vi "main_create_environment.vi"(3 "Meth. Path":refnum<vi>, 4 "Hydr. Path":refnum<vi>, 5 "Ready?":refnum<vi>, 6 "Storage?":refnum<vi>, 7 "Methane?":refnum<vi>, 8 "Running?":refnum<vi>, 9 "Directory":refnum<vi>, 10 "Create":refnum<vi>, 11 "Environtment Tree":refnum<vi>) -> ()   [LabVIEW 2019]
uses:
  lib/libSimulationControl/libSimulationControl.lvlib
panel:
  # "*******************************************************************\nBiogas Plant Control\n\nAuthor: Paul Zügel\nGCSC-Frankfurt am Main 2020\n\n*******************************************************************"
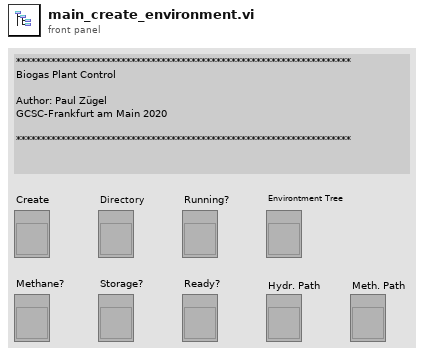
[diagram p1: front panel]
types:
  T1 = cluster{"filename without extension":string, "Child Text":string[], "Child Tag":string, i32, "Child Only?":bool, "Glyph Index":i32}[]
  T2 = enum8{"Enabled", "Disabled", "Disabled and Grayed Out"}
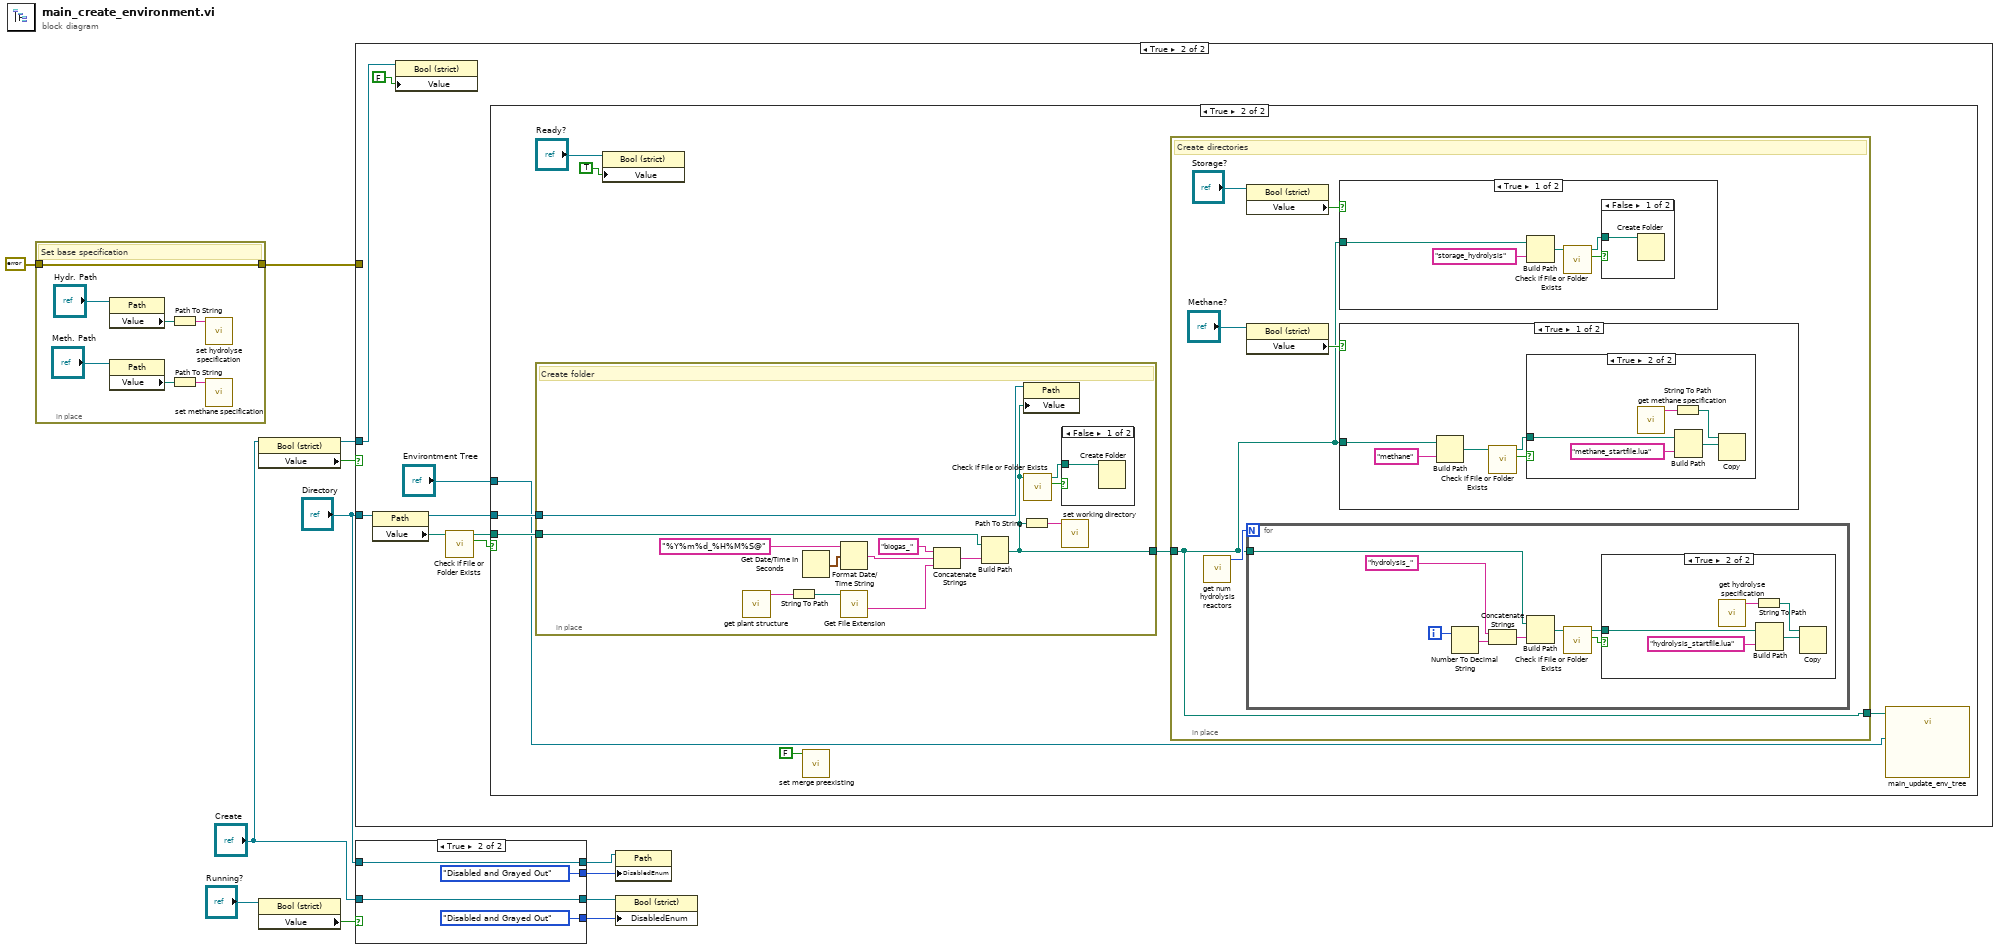
[diagram p0: block diagram]
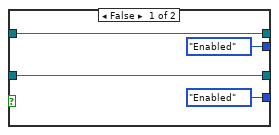
[diagram p2: hidden frame]
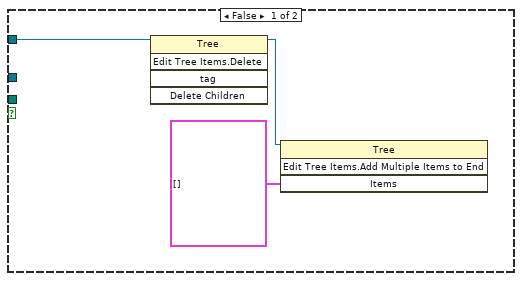
[diagram p4: hidden frame]
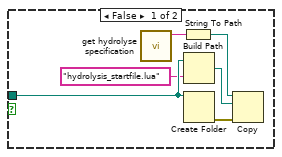
[diagram p6: hidden frame]
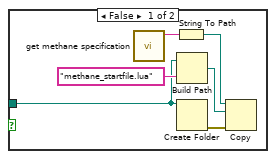
[diagram p7: hidden frame]
diagram:
  n1 = in-place {
    in-place-border: errorcluster {"status"=FALSE, "code"=0, "source"=""} ("error constant") -> [w13]
    in-place-border: [w13] -> w1
    # "Set base specification"
    n2 = property class="Path"(reference="Hydr. Path") -> ("Value"=w15:path)  [unwired: 1 in, 2 out]
    n3 = property class="Path"(reference="Meth. Path") -> ("Value"=w18:path)  [unwired: 1 in, 2 out]
    n4 = Path To String(path=w15) -> (string=w14:string)
    n5 = Path To String(path=w18) -> (string=w17:string)
    n6 = call "set hydrolyse specification.vi"("hydrolyse_spec_file"=w14) -> ()  [unwired: 10 in, 1 out]
    n7 = call "set methane specification.vi"("methane_spec_file"=w17) -> ()  [unwired: 10 in, 1 out]
  }
  n8 = property class="Bool (strict)"(reference="Create") -> (reference out=w11:refnum<vi>, "Value"=w12:bool)  [unwired: 1 in, 1 out]
  n9 = property on="Property Node" class="Bool (strict)"(reference="Running?") -> ("Value"=w9:bool)  [unwired: 1 in, 2 out]
  n10 = case shown="True" w12 {
    tunnel: w11 -> [_ w24]
    tunnel: "Directory" -> [_ w22]
    tunnel: w1 -> [_ _]
    frame False {
    }
    frame True {
      n11 = property class="Path"(reference=w22) -> (reference out=w21:refnum<vi>, "Value"=w25:path)  [unwired: 1 in, 1 out]
      n12 = property class="Bool (strict)"(reference=w24, "Value"=FALSE) -> ()  [unwired: 1 in, 2 out]
      n13 = call <vilib>:"Check if File or Folder Exists.vi"("path"=w25) -> ("file or folder exists?"=w27:bool, "dup path"=w26:path)  [unwired: 8 in, 1 out]
      n14 = case shown="True" w27 {
        tunnel: w26 -> [_ w38]
        tunnel: w21 -> [_ w34]
        tunnel: "Environtment Tree" -> [w28 w31]
        frame False {
          n15 = invoke class="Tree" method="Edit Tree Items.Delete"(reference=w28) -> (reference out=w29:refnum<vi>)  [unwired: 4 in, 4 out]
          n16 = invoke on="Invoke Node" class="Tree" method="Edit Tree Items.Add Multiple Items to End"(reference=w29, "Items"=T1 []) -> ()  [unwired: 2 in, 4 out]
        }
        frame True {
          n17 = in-place {
            in-place-border: w38 -> [w49]
            in-place-border: [w44] -> w37
            in-place-border: w34 -> [w45]
            # "Create folder"
            n18 = call "get plant structure.vi"() -> ("function return"=w47:string)  [unwired: 10 in, 1 out]
            n19 = String To Path(string=w47) -> (path=w46:path)
            n20 = Get Date/Time In Seconds() -> (seconds since 1Jan1904=w43:timestamp)
            n21 = Format Date/Time String(time format string (%c)="%Y%m%d_%H%M%S@", seconds (now)=w43) -> (date/time string=w40:string)  [unwired: 1 in]
            n22 = call <vilib>:"Get File Extension.vi"("file"=w46) -> ("filename without extension"=w39:string)  [unwired: 6 in, 4 out]
            n23 = Concatenate Strings("biogas_" ("string"), w40, w39) -> (w48:string)
            n24 = Build Path(base path=w49, name or relative path=w48) -> (appended path=w44:path)
            n25 = Path To String(path=w44) -> (string=w50:string)
            n26 = property class="Path"(reference=w45, "Value"=w44) -> ()  [unwired: 1 in, 2 out]
            n27 = call <vilib>:"Check if File or Folder Exists.vi"("path"=w44) -> ("file or folder exists?"=w52:bool, "dup path"=w51:path)  [unwired: 8 in, 1 out]
            n28 = case shown="False" w52 {
              tunnel: w51 -> [w53 _]
              frame False {
                n29 = Create Folder(path (use dialog)=w53) -> ()  [unwired: 2 in, 3 out]
              }
              frame True {
              }
            }
            n30 = call "set working directory.vi"("dir"=w50) -> ()  [unwired: 10 in, 1 out]
          }
          n31 = property class="Bool (strict)"(reference="Ready?", "Value"=TRUE) -> ()  [unwired: 1 in, 2 out]
          n32 = call "set merge preexisting.vi"("merge"=FALSE) -> ()  [unwired: 10 in, 1 out]
          n33 = in-place {
            in-place-border: w37 -> [w54]
            in-place-border: [w54] -> w32
            # "Create directories"
            n34 = call "get num hydrolysis reactors.vi"() -> ("function return"=w55:i32)  [unwired: 10 in, 1 out]
            n35 = property class="Bool (strict)"(reference="Storage?") -> ("Value"=w57:bool)  [unwired: 1 in, 2 out]
            n36 = property class="Bool (strict)"(reference="Methane?") -> ("Value"=w56:bool)  [unwired: 1 in, 2 out]
            n37 = for {
              N: w55 -> [_]
              tunnel: w54 -> [w67]
              i -> [w66]
              n38 = Number To Decimal String(number=w66) -> (decimal integer string=w60:string)  [unwired: 1 in]
              n39 = Concatenate Strings("hydrolysis_" ("string"), w60) -> (w61:string)
              n40 = Build Path(base path=w67, name or relative path=w61) -> (appended path=w65:path)
              n41 = call <vilib>:"Check if File or Folder Exists.vi"("path"=w65) -> ("file or folder exists?"=w64:bool, "dup path"=w63:path)  [unwired: 8 in, 1 out]
              n42 = case shown="True" w64 {
                tunnel: w63 -> [w70 w74]
                frame False {
                  n43 = call "get hydrolyse specification.vi"() -> ("function return"=w73:string)  [unwired: 10 in, 1 out]
                  n44 = String To Path(string=w73) -> (path=w71:path)
                  n45 = Build Path(base path=w70, name or relative path="hydrolysis_startfile.lua") -> (appended path=w68:path)
                  n46 = Create Folder(path (use dialog)=w70) -> (error out=w72:errorcluster)  [unwired: 2 in, 2 out]
                  n47 = Copy(8:w72, 10:w68, 11:w71) -> ()  [unwired: 2 in, 3 out]
                }
                frame True {
                  n48 = call "get hydrolyse specification.vi"() -> ("function return"=w78:string)  [unwired: 10 in, 1 out]
                  n49 = String To Path(string=w78) -> (path=w77:path)
                  n50 = Build Path(base path=w74, name or relative path="hydrolysis_startfile.lua") -> (appended path=w75:path)
                  n51 = Copy(10:w75, 11:w77) -> ()  [unwired: 3 in, 3 out]
                }
              }
            }
            n52 = case shown="True" w57 {
              tunnel: w54 -> [w99 _]
              frame True {
                n53 = Build Path(base path=w99, name or relative path="storage_hydrolysis") -> (appended path=w97:path)
                n54 = call <vilib>:"Check if File or Folder Exists.vi"("path"=w97) -> ("file or folder exists?"=w96:bool, "dup path"=w95:path)  [unwired: 8 in, 1 out]
                n55 = case shown="False" w96 {
                  tunnel: w95 -> [w100 _]
                  frame False {
                    n56 = Create Folder(path (use dialog)=w100) -> ()  [unwired: 2 in, 3 out]
                  }
                  frame True {
                  }
                }
              }
              frame False {
              }
            }
            n57 = case shown="True" w56 {
              tunnel: w54 -> [w83 _]
              frame True {
                n58 = Build Path(base path=w83, name or relative path="methane") -> (appended path=w81:path)
                n59 = call <vilib>:"Check if File or Folder Exists.vi"("path"=w81) -> ("file or folder exists?"=w80:bool, "dup path"=w79:path)  [unwired: 8 in, 1 out]
                n60 = case shown="True" w80 {
                  tunnel: w79 -> [w84 w92]
                  frame False {
                    n61 = call "get methane specification.vi"() -> ("function return"=w89:string)  [unwired: 10 in, 1 out]
                    n62 = String To Path(string=w89) -> (path=w87:path)
                    n63 = Build Path(base path=w84, name or relative path="methane_startfile.lua") -> (appended path=w88:path)
                    n64 = Create Folder(path (use dialog)=w84) -> (error out=w85:errorcluster)  [unwired: 2 in, 2 out]
                    n65 = Copy(8:w85, 10:w88, 11:w87) -> ()  [unwired: 2 in, 3 out]
                  }
                  frame True {
                    n66 = call "get methane specification.vi"() -> ("function return"=w94:string)  [unwired: 10 in, 1 out]
                    n67 = String To Path(string=w94) -> (path=w91:path)
                    n68 = Build Path(base path=w92, name or relative path="methane_startfile.lua") -> (appended path=w90:path)
                    n69 = Copy(10:w90, 11:w91) -> ()  [unwired: 3 in, 3 out]
                  }
                }
              }
              frame False {
              }
            }
          }
          n70 = call "main_update_env_tree.vi"("Env. Tree"=w31, "Env_path"=w32) -> ()  [unwired: 10 in]
        }
      }
    }
  }
  n71 = case shown="True" w9 {
    tunnel: "Create" -> [w104 w108]
    tunnel: "Directory" -> [w103 w107]
    tunnel: [w104 w108] -> w6
    tunnel: [w103 w107] -> w5
    tunnel: [T2."Enabled" ("Disabled") T2."Disabled and Grayed Out" ("Disabled")] -> w4
    tunnel: [T2."Enabled" ("Disabled") T2."Disabled and Grayed Out" ("Disabled")] -> w3
    frame False {
    }
    frame True {
    }
  }
  n72 = property class="Path"(reference=w5, "DisabledEnum"=w4) -> ()  [unwired: 1 in, 2 out]
  n73 = property class="Bool (strict)"(reference=w6, "DisabledEnum"=w3) -> ()  [unwired: 1 in, 2 out]
